vi "ICM Parsing Test.vi"(10 "Data String":string, 11 "Format String":string) -> (0 "error out":errorcluster, 3 "Data Values":dbl[](array[numeric]))   [LabVIEW 2018]
doc: "ICM Parsing Test.vi\n\nThis VI provides a convenient user interface for testing ICM parsing strings.\n\nInstrument Communication Module Version 1.0\nDecember, 2020 Original Code Consulting David Thomson\n www.originalcode.com"
panel:
  in  "Close on Exit?":bool
  in  "Test":bool
  in  "Stop":bool
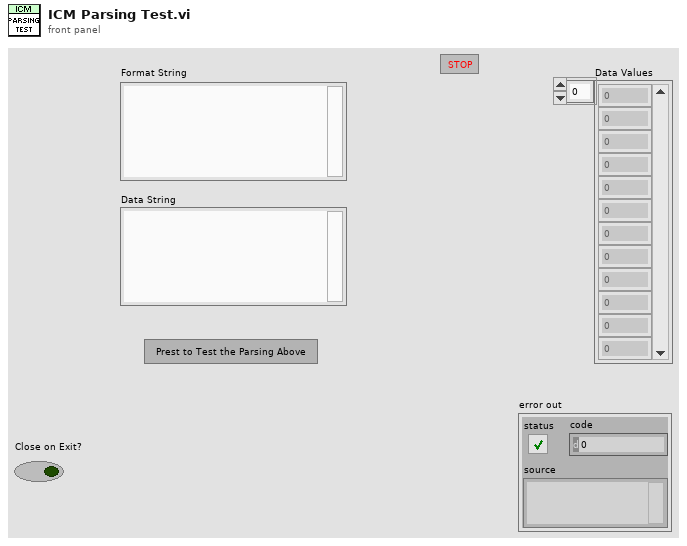
[diagram p1: front panel]
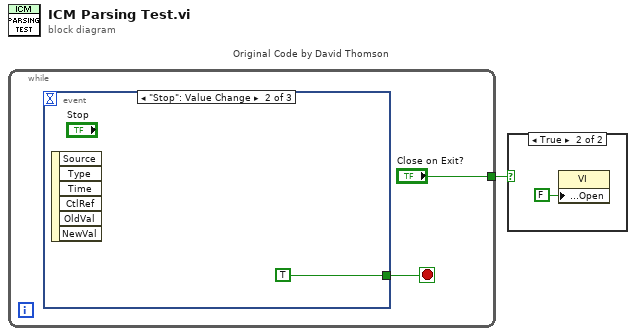
[diagram p0: block diagram]
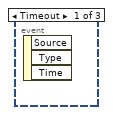
[diagram p3: hidden frame]
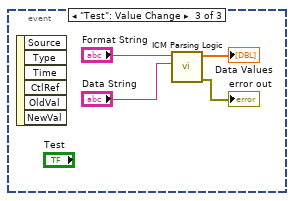
[diagram p4: hidden frame]
diagram:
  n1 = while "Original Code by David Thomson" {
    tunnel: ["Close on Exit?"] -> w1
    stop <- w3 stop-if-true
    n2 = event shown="[1] \"Stop\": Value Change" {
      selector: _ -> [_ _ _]
      dyn-events: _ -> [_ _ _]
      timeout: _ -> [_ _ _]
      tunnel: [_ TRUE _] -> w3
      event Timeout {
        n3 = event-data() -> ()  [unwired: 1 in, 3 out]
      }
      event "Stop": Value Change {
        n4 = event-data() -> ()  [unwired: 1 in, 6 out]
      }
      event "Test": Value Change {
        n5 = event-data() -> ()  [unwired: 1 in, 6 out]
        n6 = call "ICM Parsing Logic.vi"("Data String"="Data String", "Format String"="Format String") -> ("error out"=→"error out":errorcluster, "Data Values"=→"Data Values":dbl[])  [unwired: 8 in]
      }
    }
  }
  n7 = case shown="True" w1 {
    frame False {
    }
    frame True {
      n8 = property class="VI"("Front Panel.Open"=FALSE ("Front Panel Window:Open")) -> ()  [unwired: 2 in, 2 out]
    }
  }
